vi "Do Request.vi"(7 "Processing In":refnum<class "Processing.lvclass">, 11 "QueryAuthController in":refnum<class "QueryAuthController.lvclass">) -> (0 "error out":errorcluster, 5 "Processing":refnum<class "Processing.lvclass">)   [LabVIEW 2020, in "QueryAuthController.lvclass"]
uses:
  QueryAuthController.lvclass
  lv-http-util/HTTP Utils/Request/Request.lvclass
  lv-stream/stream/URI/URI.lvclass
  lv-http-util/HTTP Utils/Response/Response.lvclass
  lv-http-server/HTTP Server/Processing/Processing.lvclass
  lv-http-server/HTTP Server/Values/Values.lvclass
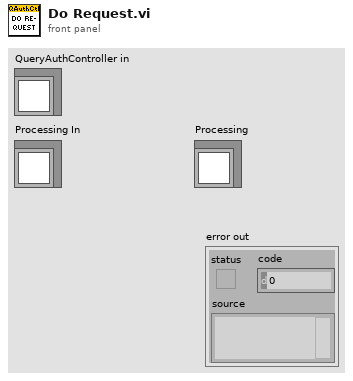
[diagram p1: front panel]
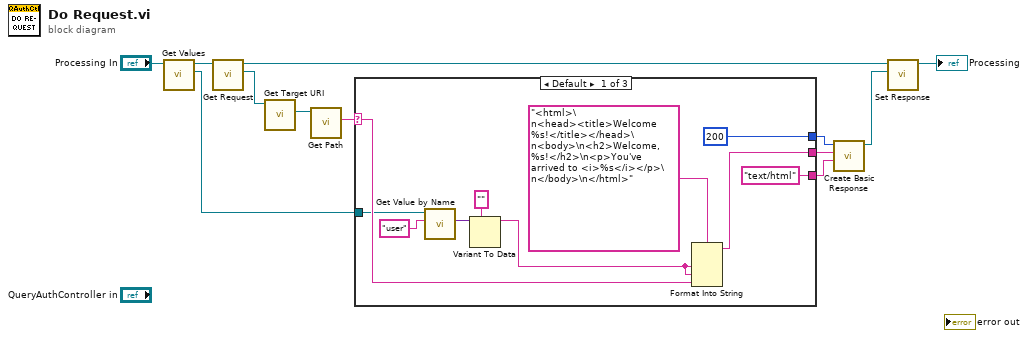
[diagram p0: block diagram]
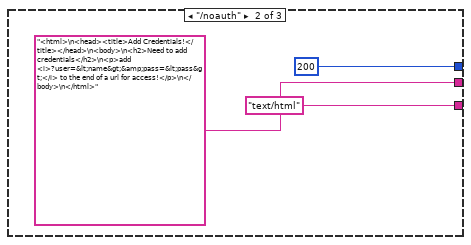
[diagram p2: hidden frame]
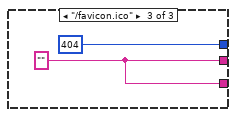
[diagram p3: hidden frame]
diagram:
  n1 = call "Get Values.vi"("Processing in"="Processing In") -> ("Values"=w5:refnum<class "Values.lvclass">, "Processing out"=w7:refnum<class "Processing.lvclass">)  [unwired: 9 in]
  n2 = call "Get Request.vi"("Processing in"=w7) -> ("Request"=w6:refnum<class "Request.lvclass">, "Processing out"=w3:refnum<class "Processing.lvclass">)  [unwired: 9 in]
  n3 = call "Get Target URI.vi"("Request in"=w6) -> ("Target URI"=w12:refnum<class "URI.lvclass">)  [unwired: 8 in, 2 out]
  n4 = call "Get Path.vi"("URI in"=w12) -> ("Path"=w11:string)  [unwired: 8 in, 2 out]
  n5 = case shown="Default" w11 {
    selector: w11 -> [w20 _ _]
    tunnel: [w22 "<html>\n<head><title>Add Credentials!</title></head>\n<body>\n<h2>Need to add credentials</h2>\n<p>add <i>?user=&lt;name&gt;&amp;pass=&lt;pass&gt;</i> to the end of a url for access!</p>\n</body>\n</html>" w26] -> w9
    tunnel: [u16 200 ("Status Code") u16 200 ("Status Code") u16 404 ("Status Code")] -> w10
    tunnel: ["text/html" "text/html" w26] -> w8
    tunnel: w5 -> [w17 _ _]
    frame Default {
      n6 = call "Get Value by Name.vi"("Name"="user" ("Name for Type (Service)"), "Values in"=w17) -> ("Value"=w15:variant)  [unwired: 7 in, 2 out]
      n7 = Variant To Data(type="", Variant=w15) -> (data=w13:string)  [unwired: 1 in, 1 out]
      n8 = Format Into String(format string="<html>\n<head><title>Welcome %s!</title></head>\n<body>\n<h2>Welcome, %s!</h2>\n<p>You've arrived to <i>%s</i></p>\n</body>\n</html>", w13, w13, w20) -> (resulting string=w22:string)  [unwired: 2 in, 1 out]
    }
    frame "/noauth" {
    }
    frame "/favicon.ico" {
      w26 = ""
    }
  }
  n9 = call "Create Basic Response.vi"("Content-Type (text/plain)"=w8, "Payload"=w9, "Status Code"=w10) -> ("Response out"=w1:refnum<class "Response.lvclass">)  [unwired: 7 in, 1 out]
  n10 = call "Set Response.vi"("Response"=w1, "Processing in"=w3) -> ("Processing out"=→"Processing":refnum<class "Processing.lvclass">)  [unwired: 9 in]
